vi "modsToOneLiner.vi"(10 "revisionNumber":string, 11 "modificationLog":string) -> (3 "oneLiner":string)   [LabVIEW 2022 SP3]
uses:
  <vilib>/Utility/error.llb/Trim Whitespace One-Sided.vi
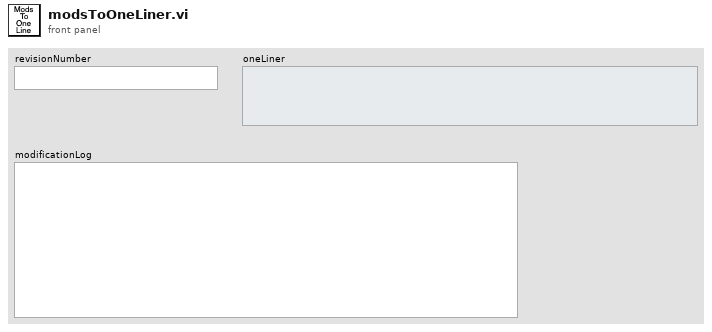
[diagram p1: front panel]
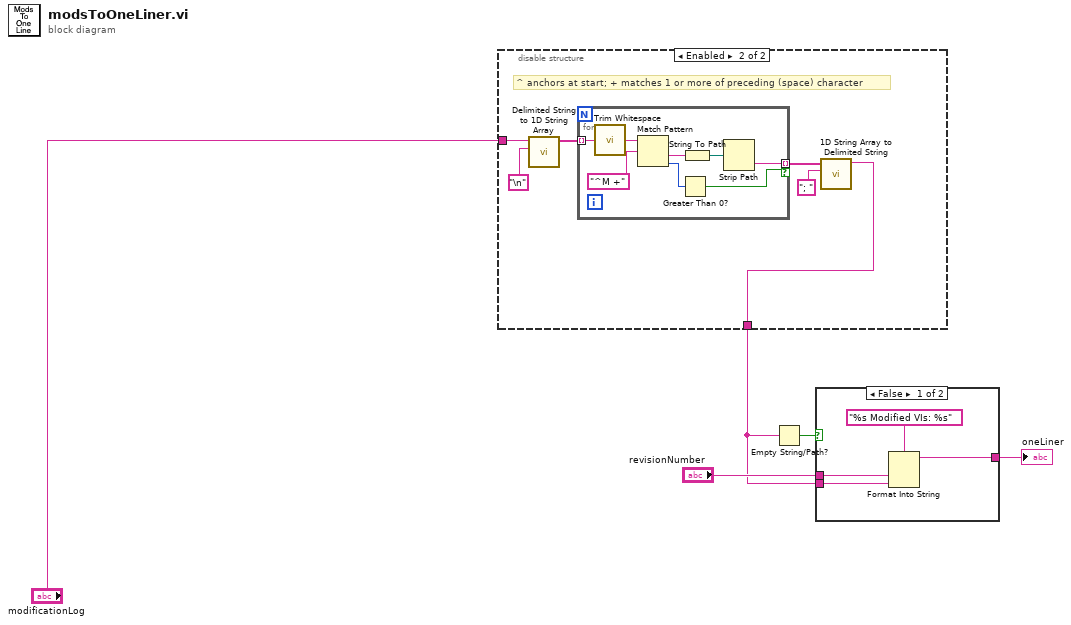
[diagram p0: block diagram]
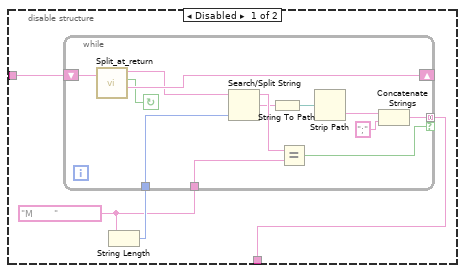
[diagram p2: hidden frame]
diagram:
  n1 = disable-structure shown="Enabled" {
    disable-tunnel: [w7 w23] -> w3
    disable-tunnel: "modificationLog" -> [w6 w24]
    frame Disabled {
      w8 = "M       "
      n2 = String Length(string=w8) -> (length=w9:i32)
      n3 = while {
        shift-right: [w21] -> _
        shift-left: w6 -> [w22]
        tunnel: w9 -> [w16]
        tunnel: w8 -> [w19]
        tunnel: [w10] -> w7 mode=concatenating if=w18
        stop <- w20 continue-if-true
        n4 = call "Split_at_return.vi"("String"=w22) -> ("before substring"=w17:string, "Matched?"=w20:bool, "after substring"=w21:string)  [unwired: 1 in, 1 out]
        n5 = Search/Split String(string=w17, offset (0)=w16) -> (substring before match=w15:string, match + rest of string=w14:string)  [unwired: 1 in, 1 out]
        n6 = String To Path(string=w14) -> (path=w13:path)
        n7 = Equal?(x=w15, y=w19) -> (x = y?=w18:bool)
        n8 = Strip Path(path=w13) -> (name=w12:string)  [unwired: 1 out]
        n9 = Concatenate Strings(w12, ";" ("string")) -> (w10:string)
      }
    }
    frame Enabled {
      # "^ anchors at start; + matches 1 or more of preceding (space) character"
      n10 = call <vilib>:"Delimited String to 1D String Array.vi"("delimiter"="\n", "delimited string"=w24) -> ("string array"=w27:string[])  [unwired: 9 in]
      n11 = for {
        tunnel: w27 -> [w36] mode=indexing
        tunnel: [w31] -> w28 mode=indexing if=w30
        n12 = call <vilib>:"Trim Whitespace.vi"("string"=w36) -> ("trimmed string"=w29:string)  [unwired: 1 in]
        n13 = Match Pattern(string=w29, regular expression="^M +") -> (after substring=w33:string, offset past match=w34:i32)  [unwired: 1 in, 2 out]
        n14 = Greater Than 0?(x=w34) -> (x > 0?=w30:bool)
        n15 = String To Path(string=w33) -> (path=w32:path)
        n16 = Strip Path(path=w32) -> (name=w31:string)  [unwired: 1 out]
      }
      n17 = call <vilib>:"1D String Array to Delimited String.vi"("delimiter"="; ", "string array"=w28) -> ("delimited string"=w23:string)  [unwired: 9 in]
    }
  }
  n18 = Empty String/Path?(string/path=w3) -> (empty?=w1:bool)
  n19 = case shown="False" w1 {
    tunnel: [w37 w41] -> w2
    tunnel: "revisionNumber" -> [w39 w41]
    tunnel: w3 -> [w38 _]
    frame False {
      n20 = Format Into String(format string="%s Modified VIs: %s", w39, w38) -> (resulting string=w37:string)  [unwired: 2 in, 1 out]
    }
    frame True {
    }
  }
  "oneLiner" <- w2
